vi "HEWH Generate Display Colors.vi"(0 "Max Temp (°F)":dbl, 1 "LV Program":T15, 5 "Min Temp (°F)":dbl, 7 "Core HEWH Data Station A":T1={"Scan Rate Adjust"=0.0, "Draw Count"=0, "Test Patten Setup"={"Total Gallons Schedule"=[], "PRAT/RLT Sequence"=[{"Sequence #"=1.0, "Cycles"=35, "Mode Setting"="", "Flow Rate (GPM)"=0.0, "Temperature (F)"=0.0, "Reset Timer"=FALSE, "Use Temp Decline Method"=FALSE, "Terminate Condition"=enum."C1-Terminate Draw @ Gallon Mark", "Condition Value #1"=0.0, "UE"=FALSE, "LE"=FALSE, "Comp"=FALSE, "Fan"=FALSE, "Test End Time (Sec)"=0.0, "Purge Until Cutout"=FALSE, "Start Conditions"=enum."Heat Source Cutout", "Condition Value #2"=0.0, "Remove Power"=FALSE, "Time"=0.0, "Check Special Cond."=enum."SC2-Check Heat Source (On-C2/Off-C1)", "Condition#"=enum."C1", "Draw Flags"=enum."N/A", "Data Processing Delay (FHD 15sec, UEF 5 Sec)"=0.0, "Test Complete"=FALSE}, {"Sequence #"=2.0, "Cycles"=15, "Mode Setting"="", "Flow Rate (GPM)"=0.0, "Temperature (F)"=0.0, "Reset Timer"=FALSE, "Use Temp Decline Method"=FALSE, "Terminate Condition"=enum."C1-Terminate Draw @ Gallon Mark", "Condition Value #1"=0.0, "UE"=FALSE, "LE"=FALSE, "Comp"=FALSE, "Fan"=FALSE, "Test End Time (Sec)"=0.0, "Purge Until Cutout"=FALSE, "Start Conditions"=enum."Heat Source Cutout", "Condition Value #2"=0.0, "Remove Power"=FALSE, "Time"=0.0, "Check Special Cond."=enum."SC2-Check Heat Source (On-C2/Off-C1)", "Condition#"=enum."C1", "Draw Flags"=enum."N/A", "Data Processing Delay (FHD 15sec, UEF 5 Sec)"=0.0, "Test Complete"=FALSE}, {"Sequence #"=3.0, "Cycles"=35, "Mode Setting"="", "Flow Rate (GPM)"=0.0, "Temperature (F)"=0.0, "Reset Timer"=FALSE, "Use Temp Decline Method"=FALSE, "Terminate Condition"=enum."C1-Terminate Draw @ Gallon Mark", "Condition Value #1"=0.0, "UE"=FALSE, "LE"=FALSE, "Comp"=FALSE, "Fan"=FALSE, "Test End Time (Sec)"=0.0, "Purge Until Cutout"=FALSE, "Start Conditions"=enum."Heat Source Cutout", "Condition Value #2"=0.0, "Remove Power"=FALSE, "Time"=0.0, "Check Special Cond."=enum."SC2-Check Heat Source (On-C2/Off-C1)", "Condition#"=enum."C1", "Draw Flags"=enum."N/A", "Data Processing Delay (FHD 15sec, UEF 5 Sec)"=0.0, "Test Complete"=FALSE}, {"Sequence #"=4.0, "Cycles"=15, "Mode Setting"="", "Flow Rate (GPM)"=0.0, "Temperature (F)"=0.0, "Reset Timer"=FALSE, "Use Temp Decline Method"=FALSE, "Terminate Condition"=enum."C1-Terminate Draw @ Gallon Mark", "Condition Value #1"=0.0, "UE"=FALSE, "LE"=FALSE, "Comp"=FALSE, "Fan"=FALSE, "Test End Time (Sec)"=0.0, "Purge Until Cutout"=FALSE, "Start Conditions"=enum."Heat Source Cutout", "Condition Value #2"=0.0, "Remove Power"=FALSE, "Time"=0.0, "Check Special Cond."=enum."SC2-Check Heat Source (On-C2/Off-C1)", "Condition#"=enum."C1", "Draw Flags"=enum."N/A", "Data Processing Delay (FHD 15sec, UEF 5 Sec)"=0.0, "Test Complete"=FALSE}, {"Sequence #"=5.0, "Cycles"=35, "Mode Setting"="", "Flow Rate (GPM)"=0.0, "Temperature (F)"=0.0, "Reset Timer"=FALSE, "Use Temp Decline Method"=FALSE, "Terminate Condition"=enum."C1-Terminate Draw @ Gallon Mark", "Condition Value #1"=0.0, "UE"=FALSE, "LE"=FALSE, "Comp"=FALSE, "Fan"=FALSE, "Test End Time (Sec)"=0.0, "Purge Until Cutout"=FALSE, "Start Conditions"=enum."Heat Source Cutout", "Condition Value #2"=0.0, "Remove Power"=FALSE, "Time"=0.0, "Check Special Cond."=enum."SC2-Check Heat Source (On-C2/Off-C1)", "Condition#"=enum."C1", "Draw Flags"=enum."N/A", "Data Processing Delay (FHD 15sec, UEF 5 Sec)"=0.0, "Test Complete"=FALSE}, {"Sequence #"=6.0, "Cycles"=15, "Mode Setting"="", "Flow Rate (GPM)"=0.0, "Temperature (F)"=0.0, "Reset Timer"=FALSE, "Use Temp Decline Method"=FALSE, "Terminate Condition"=enum."C1-Terminate Draw @ Gallon Mark", "Condition Value #1"=0.0, "UE"=FALSE, "LE"=FALSE, "Comp"=FALSE, "Fan"=FALSE, "Test End Time (Sec)"=0.0, "Purge Until Cutout"=FALSE, "Start Conditions"=enum."Heat Source Cutout", "Condition Value #2"=0.0, "Remove Power"=FALSE, "Time"=0.0, "Check Special Cond."=enum."SC2-Check Heat Source (On-C2/Off-C1)", "Condition#"=enum."C1", "Draw Flags"=enum."N/A", "Data Processing Delay (FHD 15sec, UEF 5 Sec)"=0.0, "Test Complete"=FALSE}, {"Sequence #"=7.0, "Cycles"=35, "Mode Setting"="", "Flow Rate (GPM)"=0.0, "Temperature (F)"=0.0, "Reset Timer"=FALSE, "Use Temp Decline Method"=FALSE, "Terminate Condition"=enum."C1-Terminate Draw @ Gallon Mark", "Condition Value #1"=0.0, "UE"=FALSE, "LE"=FALSE, "Comp"=FALSE, "Fan"=FALSE, "Test End Time (Sec)"=0.0, "Purge Until Cutout"=FALSE, "Start Conditions"=enum."Heat Source Cutout", "Condition Value #2"=0.0, "Remove Power"=FALSE, "Time"=0.0, "Check Special Cond."=enum."SC2-Check Heat Source (On-C2/Off-C1)", "Condition#"=enum."C1", "Draw Flags"=enum."N/A", "Data Processing Delay (FHD 15sec, UEF 5 Sec)"=0.0, "Test Complete"=FALSE}, {"Sequence #"=8.0, "Cycles"=15, "Mode Setting"="", "Flow Rate (GPM)"=0.0, "Temperature (F)"=0.0, "Reset Timer"=FALSE, "Use Temp Decline Method"=FALSE, "Terminate Condition"=enum."C1-Terminate Draw @ Gallon Mark", "Condition Value #1"=0.0, "UE"=FALSE, "LE"=FALSE, "Comp"=FALSE, "Fan"=FALSE, "Test End Time (Sec)"=0.0, "Purge Until Cutout"=FALSE, "Start Conditions"=enum."Heat Source Cutout", "Condition Value #2"=0.0, "Remove Power"=FALSE, "Time"=0.0, "Check Special Cond."=enum."SC2-Check Heat Source (On-C2/Off-C1)", "Condition#"=enum."C1", "Draw Flags"=enum."N/A", "Data Processing Delay (FHD 15sec, UEF 5 Sec)"=0.0, "Test Complete"=FALSE}], "Current Sequence Index"=0}, "HEWH Specific DAQ"={"HEWH Data"={"HEWH Standard"={"Voltage (Volts)"=0.0, "Current (Amps)"=0.0, "Power (Watts)"=0.0, "WattHours (Wh)"=0.0, "TC Tree (AVG)"=0.0, "Flow Rate (GPM)"=0.0, "Gallons (Gal)"=0.0, "RTD Out (Deg F)"=0.0, "RTD In (Deg F)"=0.0, "RTD Amb (Deg F)"=0.0, "TC Down"=0.0, "UE Event Lead"=0, "LE Event Lead"=0, "TC Tree Array"=[]}, "PRAT"={"Power (Watts) A"=4192.0, "Power (Watts) B"=4192.0, "Power (Watts) C"=4192.0, "Power (Watts) D"=4192.0, "TC1"=0.0, "TC2"=0.0, "TC3"=0.0, "TC4"=0.0, "WattHours (Wh) A"=4192.0, "WattHours (Wh) B"=4192.0, "WattHours (Wh) C"=4192.0, "WattHours (Wh) D"=4192.0, "Ambient"=0.0, "Extra Temp"=0.0}, "Additional Power Data"={"Vthd"=236.2, "Frequency (Hz)"=236.2, "Apparent Power (VA)"=236.2, "Power Factor"=236.2, "Current Crest Factor"=236.2, "Voltage Crest Factor"=236.2, "Integration Time (sec)"=236.2}}, "Flow Valve % Open"=0.0, "Power State"={"UE"=FALSE, "LE"=FALSE, "COMP"=FALSE, "FANS"=FALSE}, "Power Analyzer"=enum."APLUS", "Flow Valve uA Output"=0, "Gallons Start (Gal)"=0.0}, "Test Output Data"={"PreDraw Data Table"=[], "Data Table"=[], "MW100 TC Headers"=[]}, "Calc and Calibration"={"Mean SD Var Max Min Array"=[], "Draw Statistics (DBL)"=[], "Calibration Coefficients DBL"=[], "Start Gallons"=0.0, "Starting Temp Decline"=0.0, "K-Factor (Temperature)"=0.0, "All Draw Stats"=[], "RTD Terminate Value"=0.0, "K-Factor (Flow)"=0.0, "Intellifaucet Type"=""}, "Current Draw Time"=0.0, "LV Program"=enum."HEWH", "Station ID"=enum."A", "Current Cond"=enum."N/A", "Test Complete"=FALSE} {"Test Patten Setup"."PRAT/RLT Sequence"."Time" format="%<%H:%M:%S>t"; "Test Patten Setup"."Total Gallons Schedule" format="%.2f"}, 11 "error in (no error)":errorcluster, 12 "TC Data":string[][](array[string]), 13 "DAQ for A":bool, 14 "Station ID":string="A") -> (4 "TC Display":T17 {"TC6" format="%.2g"; "TIN" format="%.2g"; "TOUT" format="%.2g"; "TC5" format="%.2g"; "TC4" format="%.2g"; "TC3" format="%.2g"; "TC2" format="%.2g"; "TC1" format="%.2g"}, 15 "error out":errorcluster)   [LabVIEW 2016]
uses:
  Type Definitions/HEWH Tank Indicator.ctl
  Utility/Save File/File Setup (Public)/Type Definition/Save File DOE LabView Program.ctl
  Type Definitions/HEWH Output Information.ctl
  Type Definitions/HEWH Draw Pattern Setup.ctl
  Type Definitions/PRAT Test.ctl
  Utility/Save File/File Setup (Public)/Type Definition/Save File HEWH Heating Control Mode.ctl
  Draw Water Specific/Type Definitions/Terminate Draw Conditions.ctl
  Type Definitions/HEWH Start Conditions.ctl
  Draw Water Specific/Type Definitions/Check Special Condtions.ctl
  Draw Water Specific/Type Definitions/HEWH Special Condition Check.ctl
  Type Definitions/HEWH Draw Flag ENUM.ctl
  Type Definitions/HEWH Specific DAQ.ctl
  Type Definitions/HEWH Power Data.ctl
  Type Definitions/HEWH Power Elements.ctl
  Utility/Type Definitions/UTILITY Power Analyzer.ctl
  Type Definitions/HEWH Calc and Calibration.ctl
  Custom Instrument Control/MW100/Type Definitions/Station ID Selector.ctl
  Utility/Save File/File Setup.lvlib
panel:
  # "Draw Pattern Setup (24 Hour)"
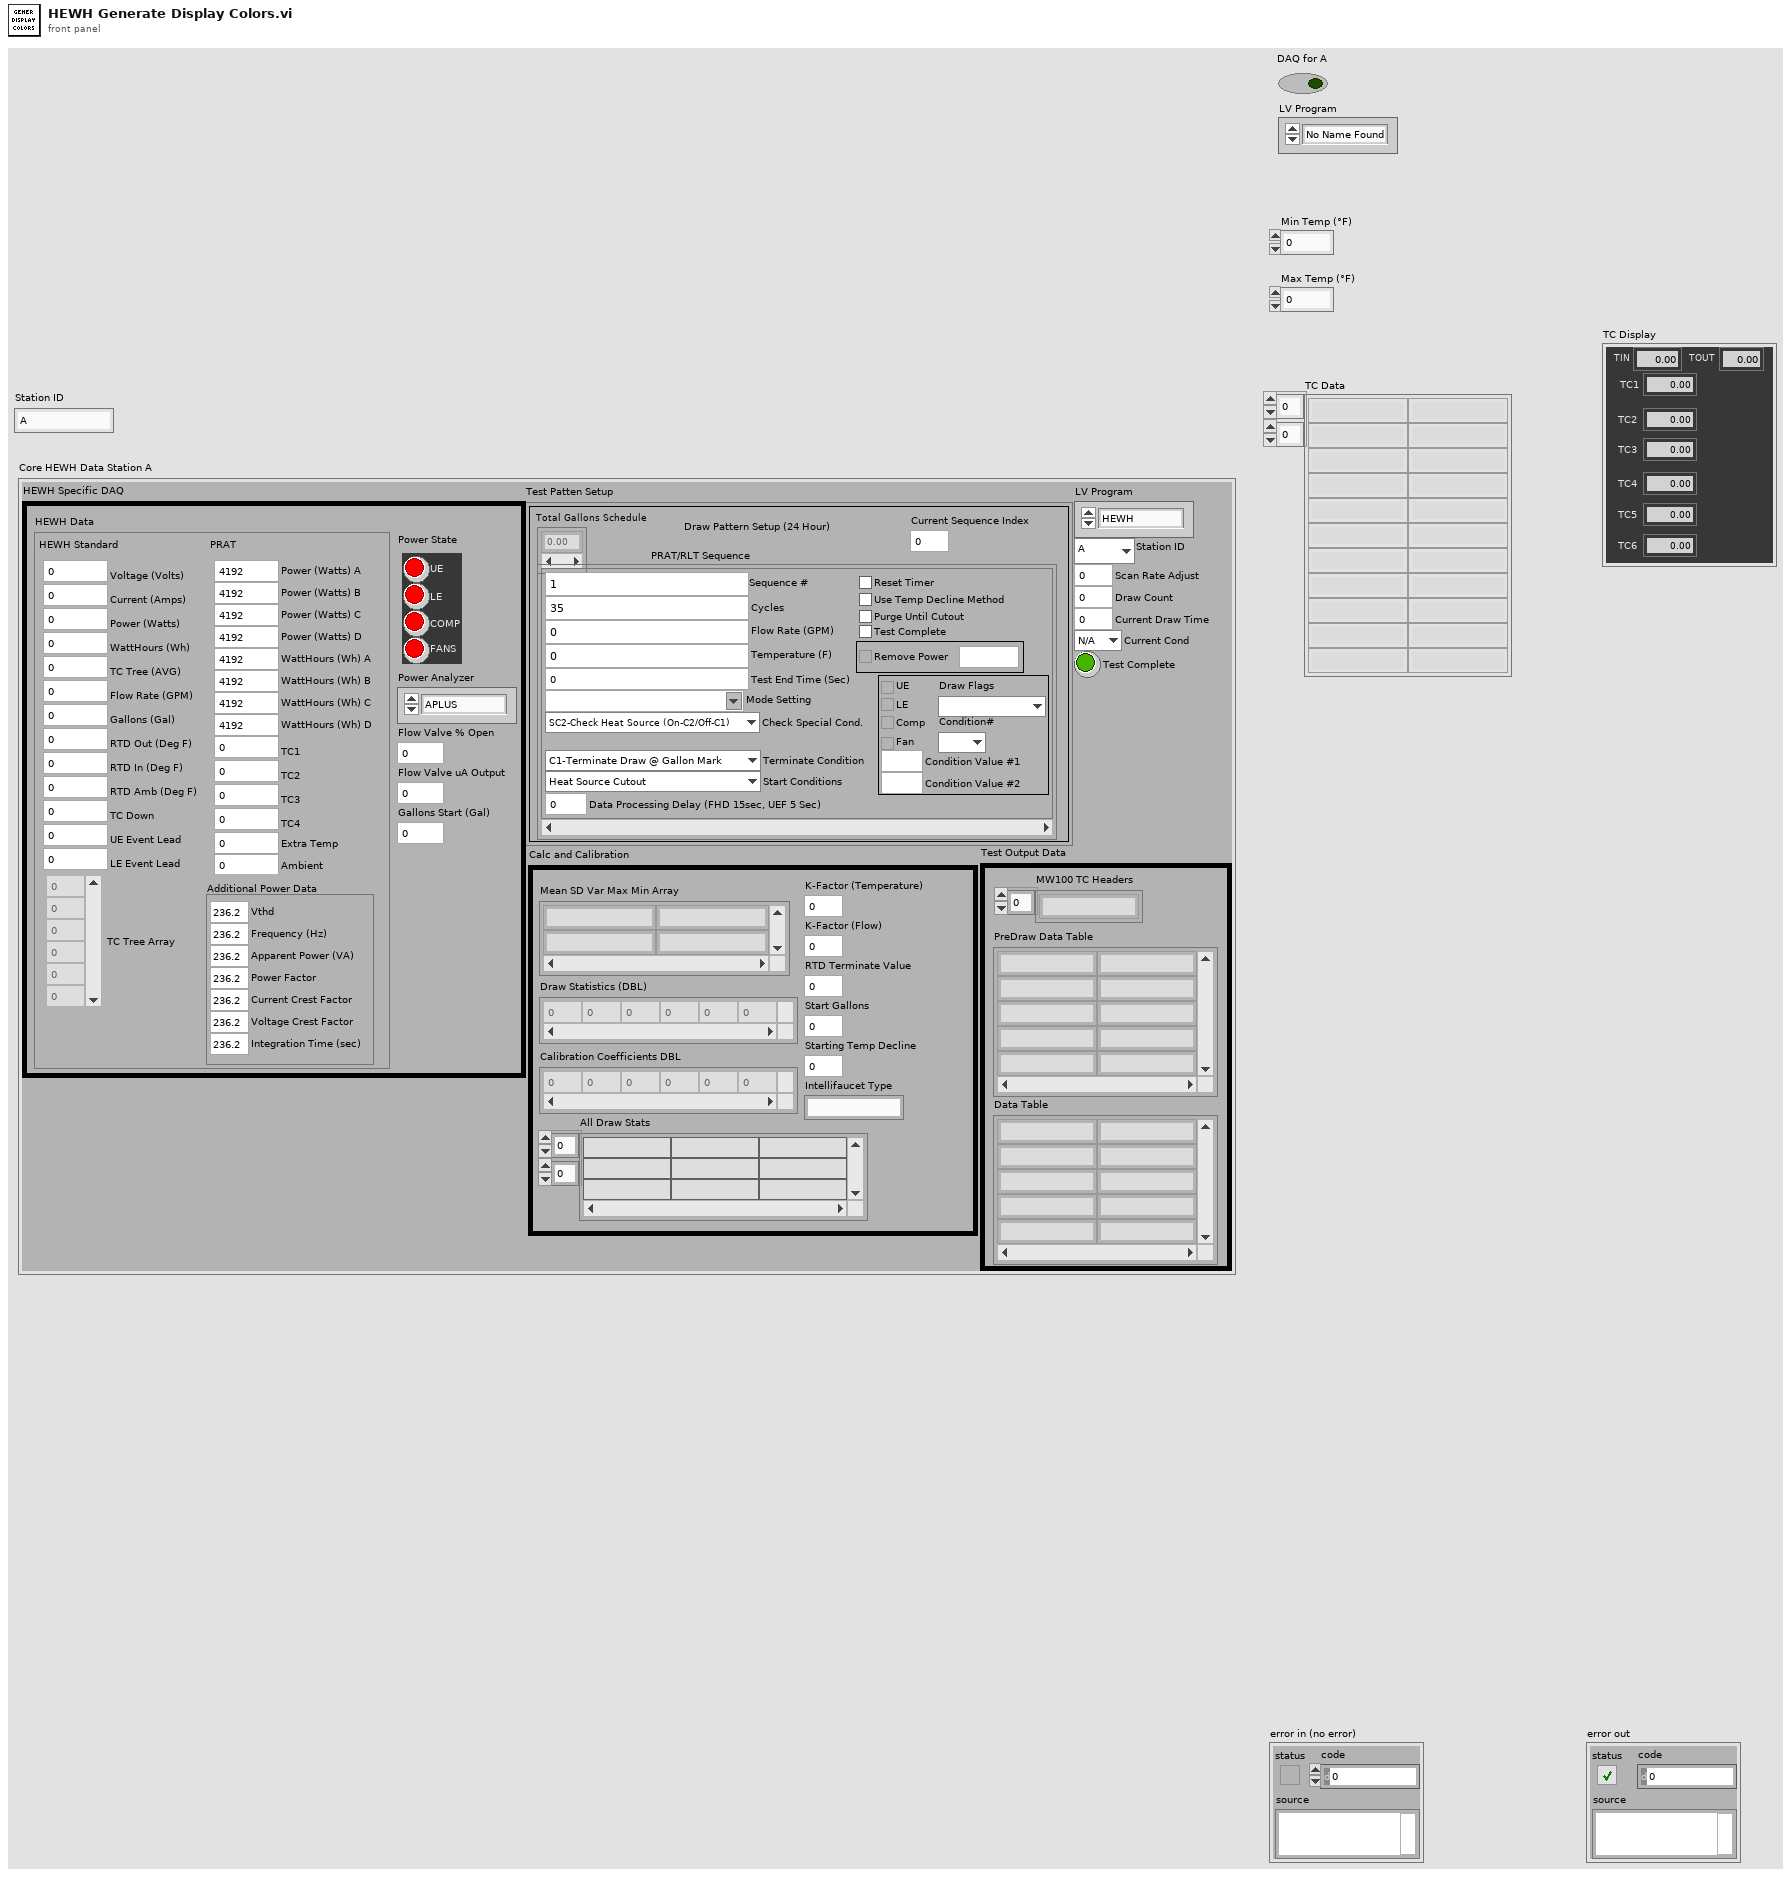
[diagram p1: front panel]
types:
  T1 = typedef "HEWH Output Information.ctl" = cluster{"Scan Rate Adjust":dbl, "Draw Count":i32, "Test Patten Setup":T2, "HEWH Specific DAQ":T10, "Test Output Data":cluster{"PreDraw Data Table":string[][], "Data Table":string[][], "MW100 TC Headers":string[]}, "Calc and Calibration":T14, "Current Draw Time":dbl, "LV Program":T15, "Station ID":T16, "Current Cond":T8, "Test Complete":bool}
  T2 = typedef "HEWH Draw Pattern Setup.ctl" = cluster{"Total Gallons Schedule":dbl[], "PRAT/RLT Sequence":T3[], "Current Sequence Index":i32}
  T3 = typedef "PRAT Test.ctl" = cluster{"Sequence #":dbl, "Cycles":i32, "Mode Setting":T4, "Flow Rate (GPM)":dbl, "Temperature (F)":dbl, "Reset Timer":bool, "Use Temp Decline Method":bool, "Terminate Condition":T5, "Condition Value #1":dbl, "UE":bool, "LE":bool, "Comp":bool, "Fan":bool, "Test End Time (Sec)":dbl, "Purge Until Cutout":bool, "Start Conditions":T6, "Condition Value #2":dbl, "Remove Power":bool, "Time":dbl, "Check Special Cond.":T7, "Condition#":T8, "Draw Flags":T9, "Data Processing Delay (FHD 15sec, UEF 5 Sec)":dbl, "Test Complete":bool}
  T4 = typedef "File Setup.lvlib/Save File HEWH Heating Control Mode.ctl" = string
  T5 = typedef "Terminate Draw Conditions.ctl" = enum16{"C1-Terminate Draw @ Gallon Mark", "C2-Special Last Draw (HU Test)", "C3-RTD Out <=", "C4-Mean Tank Temp <=", "C5-Decrease RTD Out (Deg F)", "C6-Time (Seconds)", "C7-Until Any Heat Source", "C8-Specific Heat Source", "C9-Do Nothing"}
  T6 = typedef "HEWH Start Conditions.ctl" = enum16{"Heat Source Cutout", "At Time (Seconds)", "Every X (Seconds)", "T2 >= X° Below Setpoint", "Seconds From Complete", "Wait for LE & Comp Cutout", "Wait for Comp Cutout", "Wait for LE Cutout", "Wait for UE Cutout"}
  T7 = typedef "Check Special Condtions.ctl" = enum16{"SC1-Do Nothing", "SC2-Check Heat Source (On-C2/Off-C1)", "SC3-Check Skip Condition", "SC4-Check Heat Source ON/Fail"}
  T8 = typedef "HEWH Special Condition Check.ctl" = enum16{"N/A", "C1", "C2", "Reset/Fail", "Skip Draw Sequence"}
  T9 = typedef "HEWH Draw Flag ENUM.ctl" = enum16{"N/A", "None(0)", "Sml(1)", "Med(2)", "SmlMed(3)", "Lrg(4)", "SmlLrg(5)", "MedLrg(6)", "SmlMedLrg(7)"}
  T10 = typedef "HEWH Specific DAQ.ctl" = cluster{"HEWH Data":T11, "Flow Valve % Open":dbl, "Power State":T12, "Power Analyzer":T13, "Flow Valve uA Output":i32, "Gallons Start (Gal)":dbl}
  T11 = typedef "HEWH Power Data.ctl" = cluster{"HEWH Standard":cluster{"Voltage (Volts)":dbl, "Current (Amps)":dbl, "Power (Watts)":dbl, "WattHours (Wh)":dbl, "TC Tree (AVG)":dbl, "Flow Rate (GPM)":dbl, "Gallons (Gal)":dbl, "RTD Out (Deg F)":dbl, "RTD In (Deg F)":dbl, "RTD Amb (Deg F)":dbl, "TC Down":dbl, "UE Event Lead":i32, "LE Event Lead":i32, "TC Tree Array":dbl[]}, "PRAT":cluster{"Power (Watts) A":dbl, "Power (Watts) B":dbl, "Power (Watts) C":dbl, "Power (Watts) D":dbl, "TC1":dbl, "TC2":dbl, "TC3":dbl, "TC4":dbl, "WattHours (Wh) A":dbl, "WattHours (Wh) B":dbl, "WattHours (Wh) C":dbl, "WattHours (Wh) D":dbl, "Ambient":dbl, "Extra Temp":dbl}, "Additional Power Data":cluster{"Vthd":dbl, "Frequency (Hz)":dbl, "Apparent Power (VA)":dbl, "Power Factor":dbl, "Current Crest Factor":dbl, "Voltage Crest Factor":dbl, "Integration Time (sec)":dbl}}
  T12 = typedef "HEWH Power Elements.ctl" = cluster{"UE":bool, "LE":bool, "COMP":bool, "FANS":bool}
  T13 = typedef "UTILITY Power Analyzer.ctl" = enum16{"", "APLUS", "WT210", "WT500", "WT300", "OSI", "Debug", "WT230", "WT300_1", "WT300_2"}
  T14 = typedef "HEWH Calc and Calibration.ctl" = cluster{"Mean SD Var Max Min Array":string[][], "Draw Statistics (DBL)":dbl[][], "Calibration Coefficients DBL":dbl[][], "Start Gallons":dbl, "Starting Temp Decline":dbl, "K-Factor (Temperature)":dbl, "All Draw Stats":string[][], "RTD Terminate Value":dbl, "K-Factor (Flow)":dbl, "Intellifaucet Type":string}
  T15 = typedef "File Setup.lvlib/Save File DOE LabView Program.ctl" = enum16{"No Name Found", "DOE Stand", "Dishwasher Kitchen", "Portable Stand", "HEWH", "Dryer", "Dryer WILT", "HCC", "PRAT", "HEWH RLT", "Refrigeration"}
  T16 = typedef "Station ID Selector.ctl" = enum16{"", "A", "B", "C", "D", "Global"}
  T17 = typedef "HEWH Tank Indicator.ctl" = cluster{"TC1":dbl, "TC2":dbl, "TC3":dbl, "TC4":dbl, "TC5":dbl, "TIN":dbl, "TOUT":dbl, "TC6":dbl, "TC6-Color":u32, "TC5-Color":u32, "TC4-Color":u32, "TC3-Color":u32, "TC2-Color":u32, "TC1-Color":u32, "RTD-Out":u32, "RTD-In":u32}
  T18 = typedef "HEWH Display Colors.ctl" = cluster{"Color":u32, "Temperature":dbl}
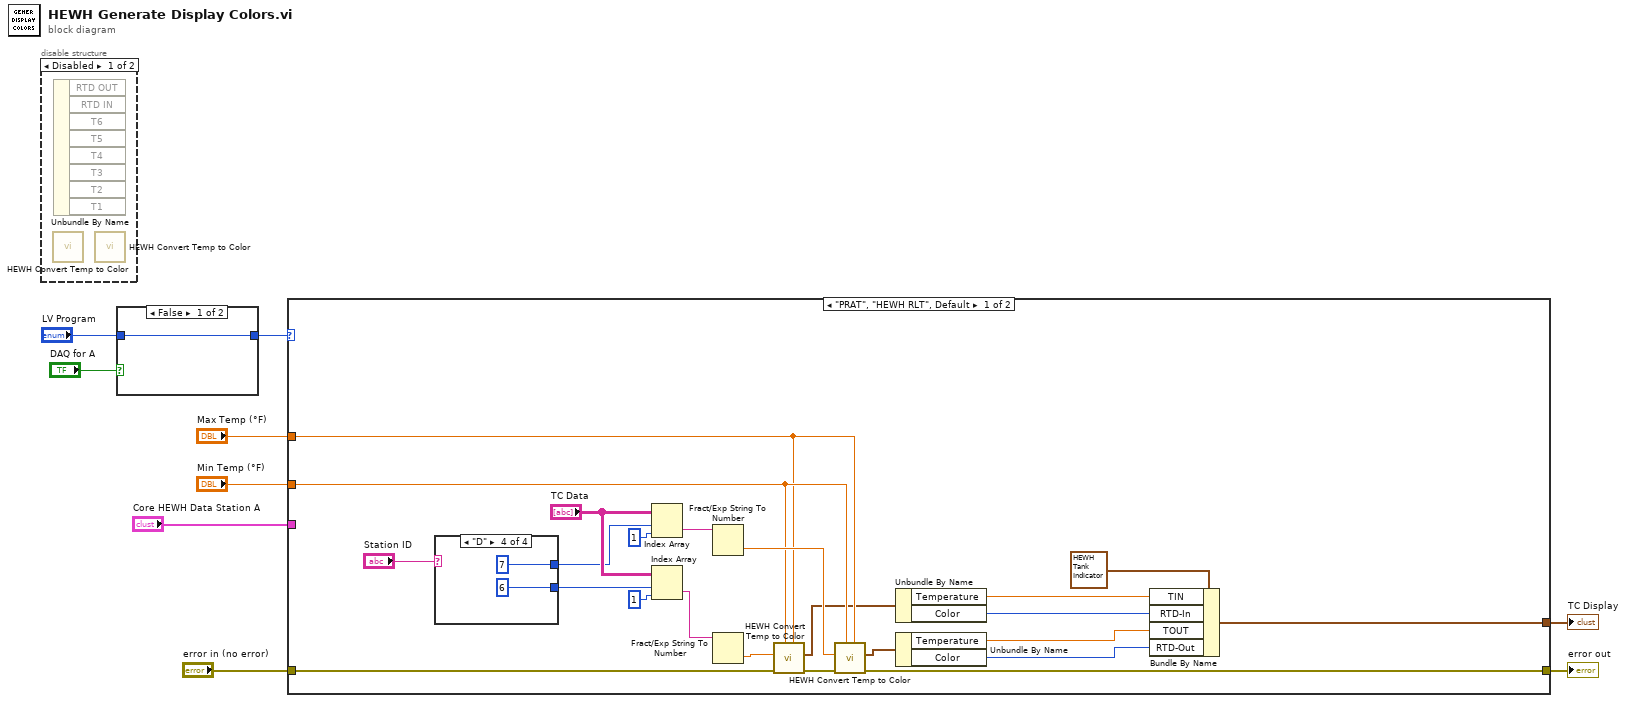
[diagram p0: block diagram]
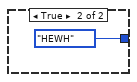
[diagram p2: hidden frame]
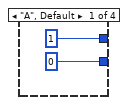
[diagram p4: hidden frame]
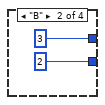
[diagram p5: hidden frame]
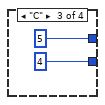
[diagram p6: hidden frame]
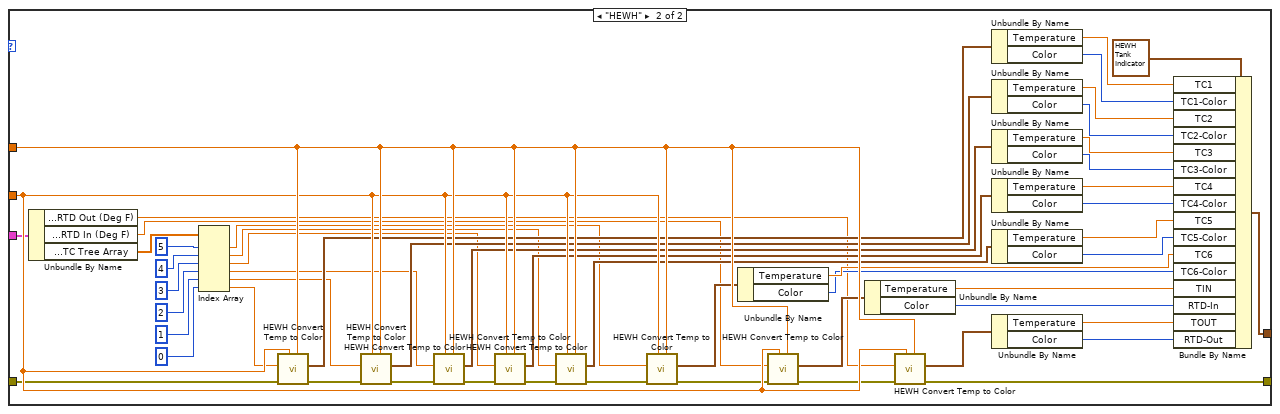
[diagram p7: hidden frame]
diagram:
  n1 = disable-structure shown="Disabled" {
    frame Disabled {
      n2 = call "HEWH Convert Temp to Color.vi"() -> ()  [unwired: 6 in, 6 out]
      n3 = Unbundle By Name() -> ()  [unwired: 1 in, 8 out]
      n4 = call "HEWH Convert Temp to Color.vi"() -> ()  [unwired: 6 in, 6 out]
    }
    frame Enabled {
    }
  }
  n5 = case shown="False" "DAQ for A" {
    tunnel: "LV Program" -> [w10 _]
    tunnel: [w10 Save_File_DOE_LabView_Program."HEWH" ("LV Program")] -> w1
    frame False {
    }
    frame True {
    }
  }
  n6 = case shown="\"PRAT\", \"HEWH RLT\", Default" w1 {
    tunnel: "Max Temp (°F)" -> [w22 w95]
    tunnel: "Min Temp (°F)" -> [w23 w94]
    tunnel: "error in (no error)" -> [w27 w93]
    tunnel: [w26 w92] -> w6
    tunnel: [w15 w83] -> w5
    tunnel: "Core HEWH Data Station A" -> [_ w51]
    frame "PRAT", "HEWH RLT", Default {
      n7 = case shown="\"D\"" "Station ID" {
        tunnel: [0 ("index (row)") 2 ("index (row)") 4 ("index (row)") 6 ("index (row)")] -> w13
        tunnel: [1 ("index (row)") 3 ("index (row)") 5 ("index (row)") 7 ("index (row)")] -> w12
        frame "A", Default {
        }
        frame "B" {
        }
        frame "C" {
        }
        frame "D" {
        }
      }
      n8 = Index Array(array="TC Data", index (row)=w12, index (col)=1 ("disabled index (col)")) -> (element=w31:string)
      n9 = Index Array(array="TC Data", index (row)=w13, index (col)=1 ("disabled index (col)")) -> (element=w30:string)
      n10 = Fract/Exp String To Number(string=w31) -> (number=w24:dbl)  [unwired: 3 in, 1 out]
      n11 = Fract/Exp String To Number(string=w30) -> (number=w25:dbl)  [unwired: 3 in, 1 out]
      n12 = call "HEWH Convert Temp to Color.vi"("Max Temp (°F)"=w22, "Min Temp (°F)"=w23, "Error In"=w27, "Temp (°F)"=w25) -> ("Error Out"=w28:errorcluster, "Control Data"=w21:T18)  [unwired: 2 in, 4 out]
      n13 = call "HEWH Convert Temp to Color.vi"("Max Temp (°F)"=w22, "Min Temp (°F)"=w23, "Error In"=w28, "Temp (°F)"=w24) -> ("Error Out"=w26:errorcluster, "Control Data"=w20:T18)  [unwired: 2 in, 4 out]
      n14 = Unbundle By Name(w21) -> ("Temperature"=w19:dbl, "Color"=w18:u32)
      n15 = Unbundle By Name(w20) -> ("Temperature"=w17:dbl, "Color"=w16:u32)
      n16 = Bundle By Name(cluster=T17 {"TC1"=0.0, "TC2"=0.0, "TC3"=0.0, "TC4"=0.0, "TC5"=0.0, "TIN"=0.0, "TOUT"=0.0, "TC6"=0.0, "TC6-Color"=0, "TC5-Color"=0, "TC4-Color"=0, "TC3-Color"=0, "TC2-Color"=0, "TC1-Color"=0, "RTD-Out"=0, "RTD-In"=0} ("Tank Display - Station A"), "TIN"=w19, "RTD-In"=w18, "TOUT"=w17, "RTD-Out"=w16) -> (w15:T17)
    }
    frame "HEWH" {
      n17 = Unbundle By Name(w51) -> ("HEWH Specific DAQ.HEWH Data.HEWH Standard.RTD Out (Deg F)"=w50:dbl, "HEWH Specific DAQ.HEWH Data.HEWH Standard.RTD In (Deg F)"=w49:dbl, "HEWH Specific DAQ.HEWH Data.HEWH Standard.TC Tree Array"=w52:dbl[])
      n18 = Index Array(array=w52, index #1=5 ("index"), index #2=4 ("index"), index #3=3 ("index"), index #4=2 ("index"), index #5=1 ("index"), index #6=0 ("index")) -> (element #1=w48:dbl, element #2=w47:dbl, element #3=w46:dbl, element #4=w45:dbl, element #5=w44:dbl, element #6=w43:dbl)
      n19 = call "HEWH Convert Temp to Color.vi"("Max Temp (°F)"=w95, "Min Temp (°F)"=w94, "Error In"=w93, "Temp (°F)"=w43) -> ("Error Out"=w85:errorcluster, "Control Data"=w82:T18)  [unwired: 2 in, 4 out]
      n20 = call "HEWH Convert Temp to Color.vi"("Max Temp (°F)"=w95, "Min Temp (°F)"=w94, "Error In"=w85, "Temp (°F)"=w44) -> ("Error Out"=w86:errorcluster, "Control Data"=w79:T18)  [unwired: 2 in, 4 out]
      n21 = call "HEWH Convert Temp to Color.vi"("Max Temp (°F)"=w95, "Min Temp (°F)"=w94, "Error In"=w86, "Temp (°F)"=w45) -> ("Error Out"=w87:errorcluster, "Control Data"=w76:T18)  [unwired: 2 in, 4 out]
      n22 = call "HEWH Convert Temp to Color.vi"("Max Temp (°F)"=w95, "Min Temp (°F)"=w94, "Error In"=w87, "Temp (°F)"=w46) -> ("Error Out"=w88:errorcluster, "Control Data"=w73:T18)  [unwired: 2 in, 4 out]
      n23 = call "HEWH Convert Temp to Color.vi"("Max Temp (°F)"=w95, "Min Temp (°F)"=w94, "Error In"=w88, "Temp (°F)"=w47) -> ("Error Out"=w89:errorcluster, "Control Data"=w70:T18)  [unwired: 2 in, 4 out]
      n24 = call "HEWH Convert Temp to Color.vi"("Max Temp (°F)"=w95, "Min Temp (°F)"=w94, "Error In"=w89, "Temp (°F)"=w48) -> ("Error Out"=w90:errorcluster, "Control Data"=w67:T18)  [unwired: 2 in, 4 out]
      n25 = Unbundle By Name(w67) -> ("Temperature"=w66:dbl, "Color"=w65:u32)
      n26 = call "HEWH Convert Temp to Color.vi"("Max Temp (°F)"=w95, "Min Temp (°F)"=w94, "Error In"=w90, "Temp (°F)"=w49) -> ("Error Out"=w91:errorcluster, "Control Data"=w64:T18)  [unwired: 2 in, 4 out]
      n27 = Unbundle By Name(w64) -> ("Temperature"=w63:dbl, "Color"=w62:u32)
      n28 = call "HEWH Convert Temp to Color.vi"("Max Temp (°F)"=w95, "Min Temp (°F)"=w94, "Error In"=w91, "Temp (°F)"=w50) -> ("Error Out"=w92:errorcluster, "Control Data"=w61:T18)  [unwired: 2 in, 4 out]
      n29 = Unbundle By Name(w82) -> ("Temperature"=w81:dbl, "Color"=w80:u32)
      n30 = Unbundle By Name(w79) -> ("Temperature"=w78:dbl, "Color"=w77:u32)
      n31 = Unbundle By Name(w76) -> ("Temperature"=w75:dbl, "Color"=w74:u32)
      n32 = Unbundle By Name(w73) -> ("Temperature"=w72:dbl, "Color"=w71:u32)
      n33 = Unbundle By Name(w70) -> ("Temperature"=w69:dbl, "Color"=w68:u32)
      n34 = Unbundle By Name(w61) -> ("Temperature"=w60:dbl, "Color"=w59:u32)
      n35 = Bundle By Name(cluster=T17 {"TC1"=95.3, "TC2"=95.2, "TC3"=95.1, "TC4"=94.5, "TC5"=91.9, "TIN"=64.4, "TOUT"=87.9, "TC6"=85.8, "TC6-Color"=4, "TC5-Color"=93, "TC4-Color"=0, "TC3-Color"=0, "TC2-Color"=0, "TC1-Color"=0, "RTD-Out"=0, "RTD-In"=4} ("Tank Display - Station A"), "TC1"=w81, "TC1-Color"=w80, "TC2"=w78, "TC2-Color"=w77, "TC3"=w75, "TC3-Color"=w74, "TC4"=w72, "TC4-Color"=w71, "TC5"=w69, "TC5-Color"=w68, "TC6"=w66, "TC6-Color"=w65, "TIN"=w63, "RTD-In"=w62, "TOUT"=w60, "RTD-Out"=w59) -> (w83:T17)
    }
  }
  "error out" <- w6
  "TC Display" <- w5
